vi "Get SCFG wrapper.vi"(8 "error in (no error)":errorcluster caption="错误输入（无错误）", 10 "dwCanNodeId":u32, 11 "dwDevIndex":u32) -> (0 "error out":errorcluster caption="错误输出", 1 "SCFG_INFO_OBJ":T1, 3 "function return":u32)   [LabVIEW 2016, in "UISimCanFunc_wrapper.lvlib"]
doc: "_declspec (dllexport) DWORD GetSCFG_wrapper(DWORD dwDevIndex, DWORD dwCanNodeId,\n P_DUMMY_SCFG_INFO_OBJ pDummySCFGInfo, P_S12CON pS12CON, P_S34CON pS34CON);"
uses:
  <userlib>/UISimCanFunc_wrapper/UISimCanFunc_wrapper.lvlib
  <userlib>/UISimCanFunc_wrapper/ctl/SCFG_INFO_OBJ.ctl
  <userlib>/UISimCanFunc_wrapper/ctl/S12CON.ctl
  <userlib>/UISimCanFunc_wrapper/ctl/S34CON.ctl
  <userlib>/UISimCanFunc_wrapper/UISimCanFunc_wrapper.dll
panel:
  in  "pS34CON":T4
  in  "pS12CON":T5
  in  "pDummySCFGInfo":cluster{"uiATCONH":u32, "uiATCONL":u32}
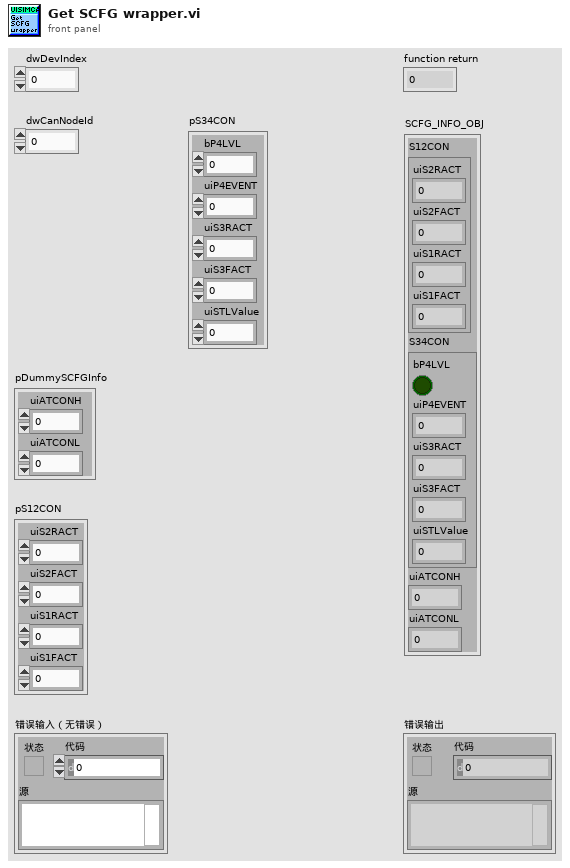
[diagram p1: front panel]
types:
  T1 = typedef "UISimCanFunc_wrapper.lvlib/SCFG_INFO_OBJ.ctl" = cluster{"S12CON":T2, "S34CON":T3, "uiATCONH":u32, "uiATCONL":u32}
  T2 = typedef "UISimCanFunc_wrapper.lvlib/S12CON.ctl" = cluster{"uiS2RACT":u32, "uiS2FACT":u32, "uiS1RACT":u32, "uiS1FACT":u32}
  T3 = typedef "UISimCanFunc_wrapper.lvlib/S34CON.ctl" = cluster{"bP4LVL":bool, "uiP4EVENT":u32, "uiS3RACT":u32, "uiS3FACT":u32, "uiSTLValue":u32}
  T4 = cluster{"bP4LVL":i32, "uiP4EVENT":u32, "uiS3RACT":u32, "uiS3FACT":u32, "uiSTLValue":u32}
  T5 = cluster{"uiS2RACT":u32, "uiS2FACT":u32, "uiS1RACT":u32, "uiS1FACT":u32}
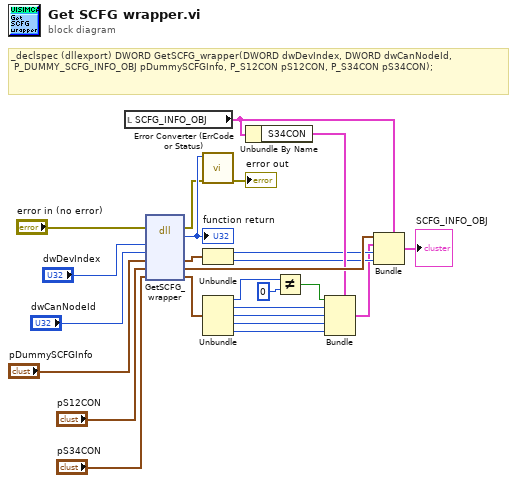
[diagram p0: block diagram]
diagram:
  # "_declspec (dllexport) DWORD GetSCFG_wrapper(DWORD dwDevIndex, DWORD dwCanNodeId,\n\tP_DUMMY_SCFG_INFO_OBJ pDummySCFGInfo, P_S12CON pS12CON, P_S34CON pS34CON);"
  n1 = local read "SCFG_INFO_OBJ"() -> (w13:T1)
  n2 = dll-call lib="C:/Program Files (x86)/National Instruments/LabVIEW 2016/user.lib/UISimCanFunc_wrapper/UISimCanFunc_wrapper.*" fn="GetSCFG_wrapper"(error in="error in (no error)", "dwDevIndex"="dwDevIndex", "dwCanNodeId"="dwCanNodeId", "pDummySCFGInfo"="pDummySCFGInfo", "pS12CON"="pS12CON", "pS34CON"="pS34CON") -> (error out=w18:errorcluster, w25:u32, "pDummySCFGInfo"=w4:cluster{"uiATCONH":u32, "uiATCONL":u32}, "pS12CON"=w15:T5, "pS34CON"=w14:T4)  [unwired: 4 in, 1 out]
  "function return" <- w25
  n3 = call <userlib>:"Error Converter (ErrCode or Status).vi"("error in (no error)"=w18, "error code"=w25) -> ("error out"=→"error out":errorcluster)  [unwired: 9 in]
  n4 = Unbundle(w4) -> ("uiATCONH"=w3:u32, "uiATCONL"=w2:u32)
  n5 = Unbundle(w14) -> ("bP4LVL"=w10:i32, "uiP4EVENT"=w8:u32, "uiS3RACT"=w7:u32, "uiS3FACT"=w6:u32, "uiSTLValue"=w5:u32)
  n6 = Unbundle By Name(w13) -> ("S34CON"=w12:T3)
  n7 = Not Equal?(x=w10, y=0) -> (x != y?=w9:bool)
  n8 = Bundle(cluster=w12, "bP4LVL"=w9, "uiP4EVENT"=w8, "uiS3RACT"=w7, "uiS3FACT"=w6, "uiSTLValue"=w5) -> (w1:T3)
  n9 = Bundle(cluster=w13, "S12CON"=w15, "S34CON"=w1, "uiATCONH"=w3, "uiATCONL"=w2) -> (→"SCFG_INFO_OBJ":T1)
